vi "FB Switch Bool Input Term Var Write.vi"(8 "error in":errorcluster, 10 "invert":bool, 11 "data in":variant) -> (0 "error out":errorcluster, 3 "data out":variant)   [LabVIEW 2020]
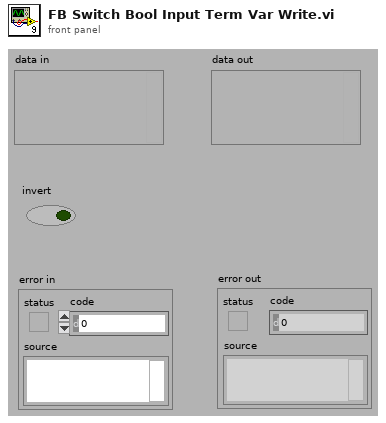
[diagram p1: front panel]
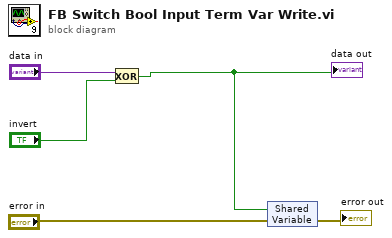
[diagram p0: block diagram]
diagram:
  n1 = Exclusive Or(1:"invert", 2:"data in") -> (0:w1:bool)
  "data out" <- w1
  n2 = shared-variable(w1, error in="error in") -> (error out=→"error out":errorcluster)
